vi "Insert View.vi"(8 "error in (no error)":errorcluster, 9 "Insertion Request Time":timestamp, 10 "Protected Subpanel":T1, 11 "IViewable in":refnum<class "IViewable.lvclass">) -> (0 "error out":errorcluster, 3 "IViewable out":refnum<class "IViewable.lvclass">)   [LabVIEW 2015, in "IViewable.lvlib" / "IViewable.lvclass"]
doc: "<License>\nCopyright © 2017 Composed Systems, LLC | All rights reserved\nwww.composed.io\n\nAuthor: Ethan Stern <ethan.stern@composed.io>\n\nThis software is provided \"AS IS\" WITHOUT WARRANTIES, either express or implied, AND IS FOR EDUCATIONAL PURPOSES ONLY.\n</License>"
uses:
  IViewable.lvclass
  <vilib>/Composed Systems/Protected Subpanel/Protected Subpanel Reference.ctl
  <vilib>/Composed Systems/Protected Subpanel/ProtectedSubpanel.lvclass
  IViewable.lvclass/IViewable.ctl
  <vilib>/Utility/LVClass/Get LV Class Name.vi
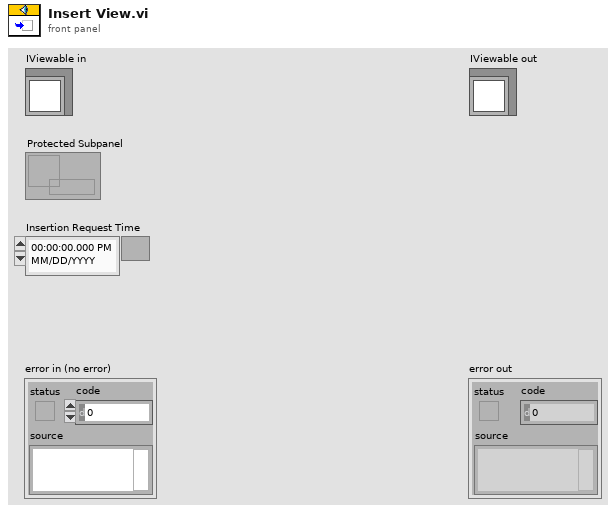
[diagram p1: front panel]
types:
  T1 = typedef "ProtectedSubpanel.lvlib/ProtectedSubpanel.lvclass/Protected Subpanel Reference.ctl" = refnum<data-value>
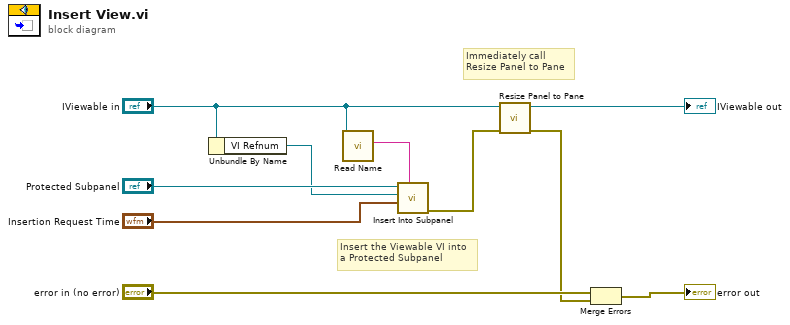
[diagram p0: block diagram]
diagram:
  # "Immediately call\nResize Panel to Pane"
  # "Insert the Viewable VI into\na Protected Subpanel"
  n1 = Unbundle By Name("IViewable in") -> ("VI Refnum"=w7:refnum<vi>)
  n2 = call "Read Name.vi"("IViewable In"="IViewable in") -> ("Name"=w4:string)  [unwired: 8 in, 2 out]
  n3 = call <vilib>:"Insert Into Subpanel.vi"("Viewable Name"=w4, "Insertion Request Time"="Insertion Request Time", "VI Refnum"=w7, "Protected Subpanel"="Protected Subpanel") -> ("error out"=w2:errorcluster)  [unwired: 6 in, 1 out]
  n4 = call-dynamic "Resize Panel to Pane.vi"("error in (no error)"=w2, "IViewable In"="IViewable in") -> ("error out"=w1:errorcluster, "IViewable Out"=→"IViewable out":refnum<class "IViewable.lvclass">)  [unwired: 8 in]
  n5 = Merge Errors("error in (no error)", w1) -> (→"error out":errorcluster)
